vi "Watch_Directory.vi"() -> ()   [LabVIEW 2015]
uses:
  <userlib>/caLab/Private/Get_PV-1D.vi
panel:
  in  "string 2":string="P:\\bl13-0\\bl13-2\\dt_SES100\\"
  in  "OK Button":bool
  in  "ELOG":string
  out "path":path
  in  "Subdir":string
  out "file path 2":path=path "S:/"
  in  "Ring":u16(ring) items=["SES-100", "R3000"]
  out "spreadsheet string":string
  out "PV Names (dup)":string[](array[string])
  out "PV2ELOG":string
  out "concatenated string":string
  out "standard error":string
  out "standard output":string
  out "x = y?":bool
  out "File Name 1":string
  in  "Filter":string
  in  "stop":bool
  out "File Name 0":string
  in  "Path":path=path "D:/Documents and Settings/Customer Education/My Documents"
  # "Set a folder to watch using the\nPath control. You can also\nset a filter for a certain type\nof file to watch for (such as\n*.bmp). Then run the\nexample. Whenever you create\na new file in that directory that\nmatches the filter, New File Name\nwill update to let you know the\nnew file name."
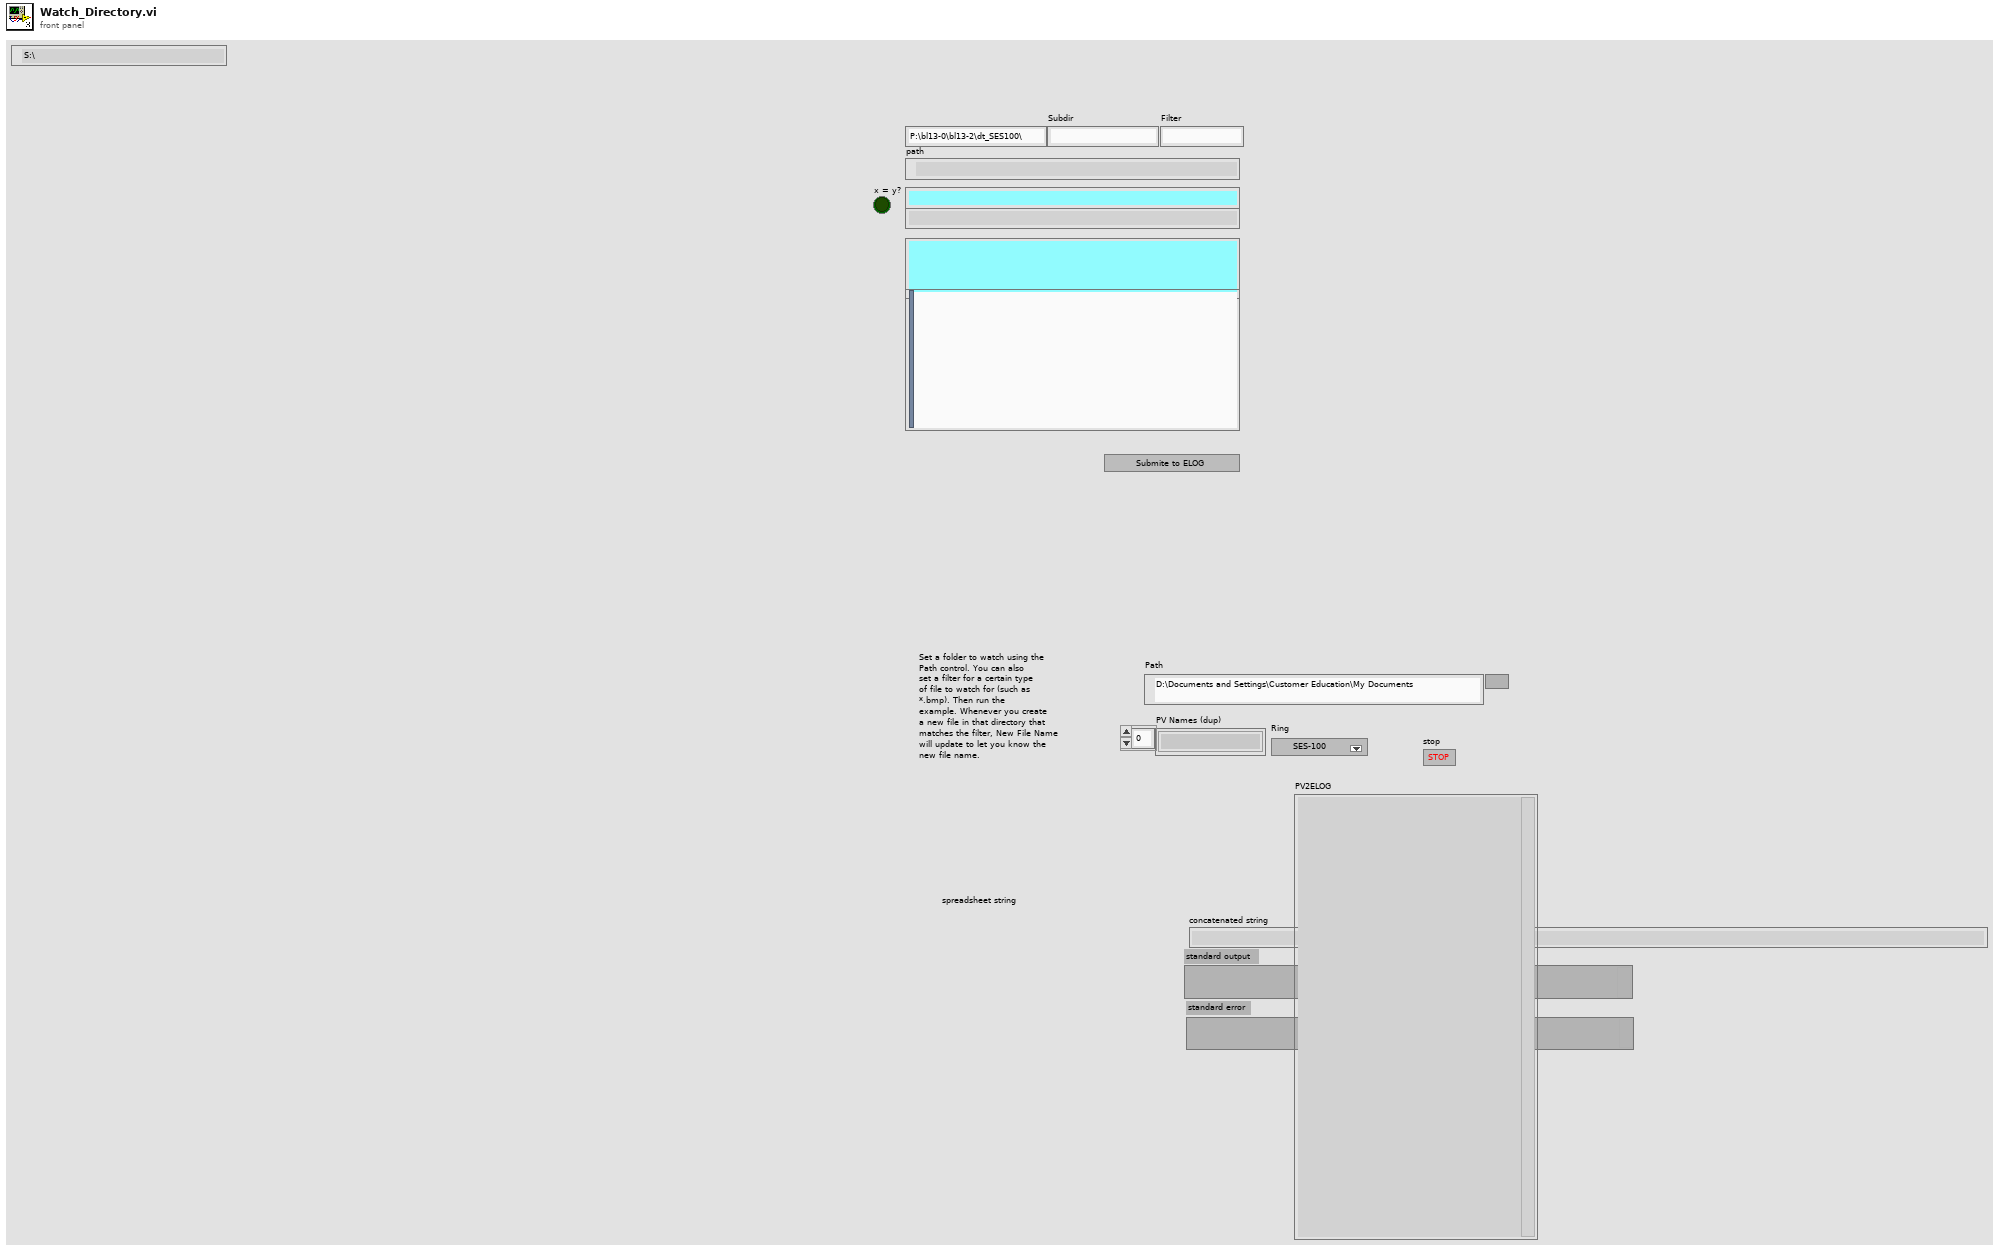
[diagram p1: front panel]
types:
  T1 = enum16{"open", "replace", "create", "open or create", "replace or create", "replace or create with confirmation"}
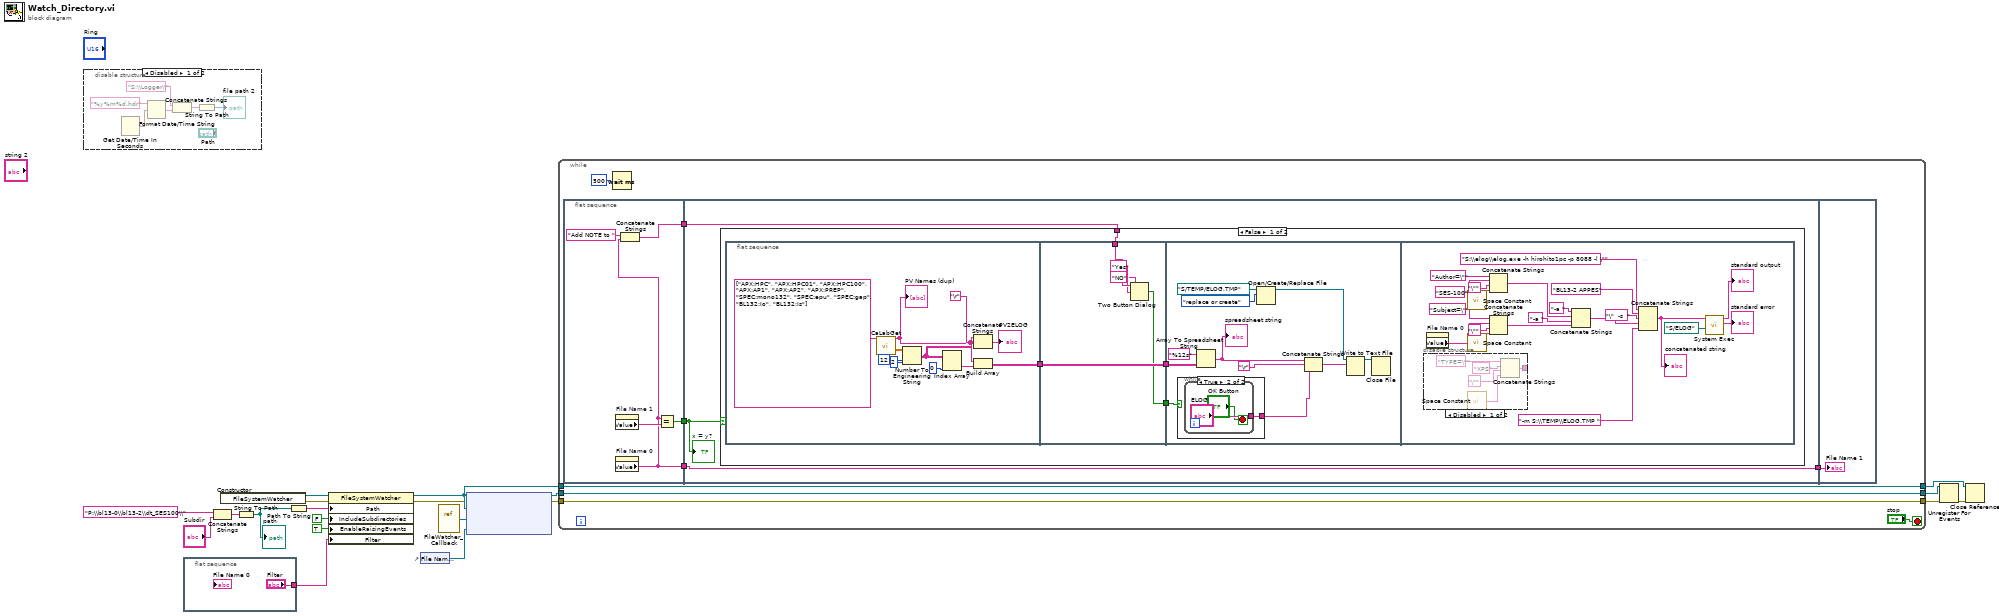
[diagram p0: block diagram]
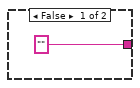
[diagram p3: hidden frame]
diagram:
  n1 = disable-structure shown="Disabled" {
    frame Disabled {
      n2 = Get Date/Time In Seconds() -> (seconds since 1Jan1904=w26:timestamp)
      n3 = Format Date/Time String(time format string (%c)="%y%m%d.hdr", seconds (now)=w26) -> (date/time string=w23:string)  [unwired: 1 in]
      n4 = Concatenate Strings("S:\\Logger\\", w23) -> (w22:string)
      n5 = String To Path(string=w22) -> (path=→"file path 2":path)
    }
    frame Enabled {
    }
  }
  n6 = flat-sequence {
    tunnel: ["Filter"] -> w6
    frame #0 {
    }
  }
  n7 = Concatenate Strings("P:\\bl13-0\\bl13-2\\dt_SES100\\" ("string"), "Subdir") -> (w2:string)
  n8 = constructor class="FileSystemWatcher"() -> (reference out=w20:refnum<k24>, error out=w11:errorcluster)  [unwired: 3 in, 1 out]
  n9 = String To Path(string=w2) -> (path=w1:path)
  "path" <- w1
  n10 = Path To String(path=w1) -> (string=w19:string)
  n11 = property class="FileSystemWatcher"(reference=w20, error in=w11, "Path"=w19, "IncludeSubdirectories"=FALSE, "EnableRaisingEvents"=TRUE, "Filter"=w6) -> (reference out=w14:refnum<k24>, error out=w10:errorcluster)
  n12 = control-ref of="File Name 0"() -> (w5:refnum<vi>)
  n13 = vi-ref "FileWatcher_Callback.vi"() -> ("vi reference"=w17:refnum<vi>)
  n14 = node(w10, w14, w17, w5) -> (w15:refnum<k27>, w8:errorcluster)  [unwired: 1 in]
  n15 = while {
    tunnel: [w35] -> w16
    tunnel: w15 -> [w35]
    tunnel: [w34] -> w12
    tunnel: w14 -> [w34]
    tunnel: [w33] -> w9
    tunnel: w8 -> [w33]
    stop <- "stop" stop-if-true
    n16 = flat-sequence {
      tunnel: [w38] -> w31
      tunnel: [w40] -> w29
      tunnel: [w37] -> w28
      tunnel: w31 -> [w44]
      tunnel: [w44] -> w30
      tunnel: w29 -> [w43]
      tunnel: w28 -> [w42]
      tunnel: w30 -> [w106]
      frame #0 {
        n17 = property on="File Name 1" class="Str"() -> ("Value"=w41:string)  [unwired: 2 in, 2 out]
        n18 = property on="File Name 0" class="Str"() -> ("Value"=w38:string)  [unwired: 2 in, 2 out]
        n19 = Concatenate Strings("Add NOTE to " ("string"), w38) -> (w37:string)
        n20 = Equal?(x=w38, y=w41) -> (x = y?=w40:bool)
      }
      frame #1 {
        n21 = case shown="False" w43 {
          tunnel: w42 -> [w46 _]
          frame False {
            n22 = flat-sequence {
              tunnel: [w51] -> w47
              tunnel: [w64] -> w48
              tunnel: w47 -> [w64]
              tunnel: w46 -> [w63]
              tunnel: [w60] -> w45
              tunnel: w48 -> [w70]
              tunnel: w45 -> [w65]
              frame #0 {
                n23 = call-poly <userlib>:"CaLabGet.vi"("PV Names"=string[] ["APX:HPC", "APX:HPC01", "APX:HPC100", "APX:AP1", "APX:AP2", "APX:PREP", "SPEC:mono132", "SPEC:epu", "SPEC:gap", "BL132:Io", "BL132:Is"]) -> ("PV Names (dup)"=w55:string[], "Value Array (number)"=w57:dbl[][])  [unwired: 8 in, 5 out]
                "PV Names (dup)" <- w55
                n24 = Number To Engineering String(2:i16 2 ("precision (6)"), 3:i16 12 ("width (-)"), 4:w57) -> (0:w53:string[][])  [unwired: 1 in]
                n25 = Index Array(array=w53, index (col)=0) -> (element=w52:string[])  [unwired: 1 in]
                n26 = Concatenate Strings(w55, "\r", w53) -> (→"PV2ELOG":string)
                n27 = Build Array(w55, w52) -> (w51:string[][])
              }
              frame #1 {
                n28 = Two Button Dialog(message=w63, 1:"NO" ("F button name (\"Cancel\")"), 2:"Yes" ("T button name (\"OK\")")) -> (T button?=w60:bool)
              }
              frame #2 {
                n29 = case shown="True" w65 {
                  tunnel: ["" ("ELOG") w77] -> w68
                  frame False {
                  }
                  frame True {
                    n30 = while {
                      tunnel: ["ELOG"] -> w77
                      stop <- "OK Button" stop-if-true
                    }
                  }
                }
                n31 = Array To Spreadsheet String(array=w70, 3:"%12s" ("format string")) -> (spreadsheet string=w67:string)  [unwired: 1 in]
                "spreadsheet string" <- w67
                n32 = Open/Create/Replace File(file path (use dialog)=path "S:/TEMP/ELOG.TMP", operation (0:open)=T1."replace or create") -> (refnum out=w75:refnum<file>)  [unwired: 4 in, 2 out]
                n33 = Concatenate Strings(w67, "\r", w68) -> (w66:string)
                n34 = Write to Text File(file (use dialog)=w75, text=w66) -> (refnum out=w74:refnum<file>)  [unwired: 2 in, 2 out]
                n35 = Close File(refnum=w74) -> ()  [unwired: 1 in, 2 out]
              }
              frame #3 {
                n36 = disable-structure shown="Disabled" {
                  disable-tunnel: [w101 _] -> _
                  frame Disabled {
                    n37 = call <vilib>:"Space Constant.vi"() -> ("String"=w102:string)
                    n38 = Concatenate Strings("TYPE=\"" ("string"), "XPS", "\"" ("string"), w102) -> (w101:string)
                  }
                  frame Enabled {
                  }
                }
                n39 = property on="File Name 0" class="Str"() -> ("Value"=w80:string)  [unwired: 2 in, 2 out]
                n40 = call <vilib>:"Space Constant.vi"() -> ("String"=w86:string)
                n41 = call <vilib>:"Space Constant.vi"() -> ("String"=w87:string)
                n42 = Concatenate Strings("Author=\"" ("string"), "SES-100", "\"" ("string"), w86) -> (w84:string)
                n43 = Concatenate Strings("Subject=\"" ("string"), w80, "\"" ("string"), w87) -> (w82:string)
                n44 = Concatenate Strings("-a ", w84, "-a " ("string"), w82) -> (w83:string)
                n45 = Concatenate Strings("S:\\elog\\elog.exe -h hirohito1pc -p 8088 -l \"" ("command line"), "BL13-2 APPES", "\"  -s  " ("command line"), w83, "-m S:\\TEMP\\ELOG.TMP " ("string")) -> (w95:string)
                "concatenated string" <- w95
                n46 = call <vilib>:"System Exec.vi"("working directory"=path "S:/ELOG", "command line"=w95) -> ("standard error"=→"standard error":string, "standard output"=→"standard output":string)  [unwired: 6 in, 2 out]
              }
            }
          }
          frame True {
          }
        }
        "x = y?" <- w43
      }
      frame #2 {
        "File Name 1" <- w106
      }
    }
    n47 = Wait (ms)(milliseconds to wait=u32 500) -> ()  [unwired: 1 out]
  }
  n48 = Unregister For Events(event registration refnum=w16, error in=w9) -> (error out=w13:errorcluster)
  n49 = Close Reference(reference=w12, error in (no error)=w13) -> ()  [unwired: 1 out]
